vi "zlgcan_demo_EU.vi"() -> ()   [LabVIEW 2018]
doc: "适用的设备：PCI-5010-U、PCI-5020-U、USBCAN-E-U、\nUSBCAN-2E-U、USBCAN-4E-U、USBCAN-8E-U、CANalyst-II+"
uses:
  data_type/ZCAN_Transmit_Data.ctl
  data_type/ZCAN_InitCAN_setting_EU.ctl
panel:
  in  "ZCAN_InitCAN_Setting_EU":T1
  in  "开启CAN":bool
  in  "stop":bool
  in  "?":T2(tab)
  in  "CAN 通道":u32(ring) items=["0", "1"]
  in  "CAN卡型号":u32(ring)=31 items=["PCI-5010-U"=19, "PCI-5020-U"=22, "USBCAN_E_U"=20, "USBCAN_2E_U"=21, "USBCAN-4E-U"=31]
  in  "索引":u32(ring) items=["0", "1", "2", "3", "4", "5", "6", "7", "8"]
  in  "波特率":u32(ring)=500000 items=["1Mbps"=1000000, "800kbps"=800000, "500kbps"=500000, "250kbps"=250000, "125kbps"=125000, "100kbps"=100000, "50kbps"=50000]
  in  "自定义波特率？":bool
  in  "自定义波特率字符输入":string
  in  "工作模式":u8(ring) items=["正常", "只听"]
  out "设备句柄":u32
  out "通道句柄":u32
  out "error out":errorcluster caption="状态"
  in  "帧类型":u32(ring) items=["标准帧", "扩展帧"]
  in  "发送方式":u32(ring) items=["正常发送", "单次发送", "自发自收", "单次自发自收"]
  in  "帧格式":u32(ring) items=["数据帧", "远程帧"]
  out "数据长度":u8=8 max=8
  in  "ID":u32=18 format="0x%08x"
  in  "协议":u32(ring) items=["CAN"]
  in  "数据输入":string="11 22 33 44 55 66 77 88"
  in  "发送":bool
  in  "CAN数据帧数组":T3(array[cluster])
  out "CAN报文显示":string[][](table)
  in  "ZCAN_Transmit_Data":T4
  out "已接收帧数":u32
  # "适用的设备：PCI-5010-U、PCI-5020-U、USBCAN-E-U、\nUSBCAN-2E-U、USBCAN-4E-U"
  # "停止程序前，请先关闭CAN卡"
  # "1. 确保电脑有VC++ 2005/2008/2010/2013运行库（对应32，64位）,微软常用运行库合集，点击下载（35M）。\n    http://manual.zlg.cn/Public/Uploads/2020-06-05/5ed995c271414.zip"
  # "2，如果打开设备失败，可能原因：\n（1）已经打开过一次，没有正常关闭的情况下，继续点击“打开设备”，是无法打开的。\n     需要USB重新拔插，LABVIEW重启（全部关闭），然后再“打开设备”。\n (2) 项目路径不能有中文繁体。"
  # "使用ZCANPro软件波特率计算工具计算"
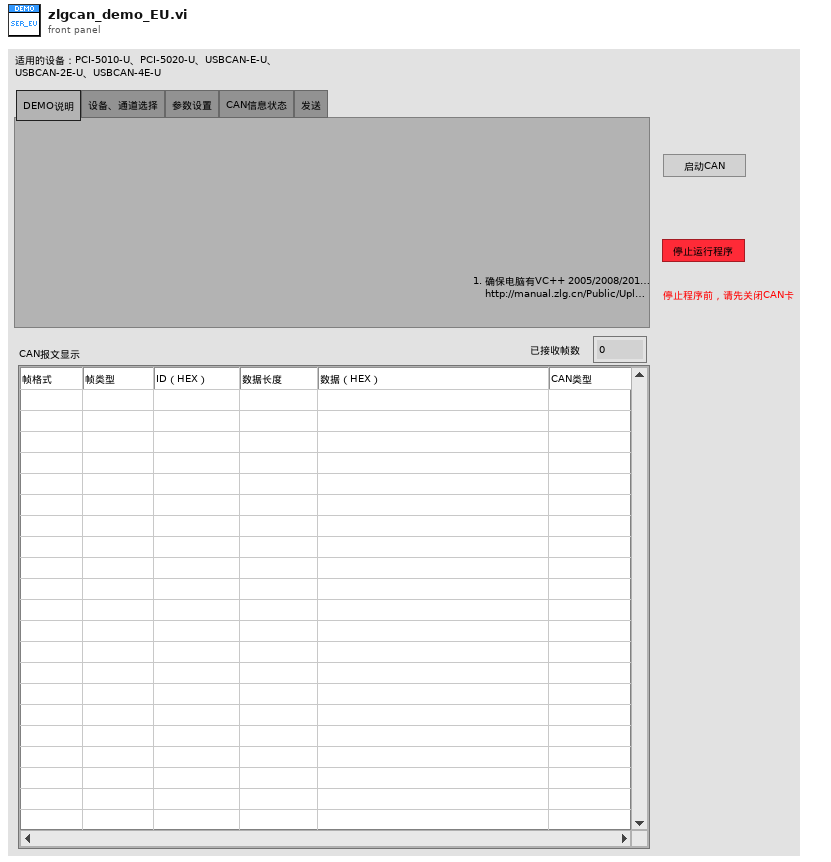
[diagram p1: front panel]
types:
  T1 = typedef "ZCAN_InitCAN_setting_EU.ctl" = cluster{"baudrate":u32, "baud_rate_custom？":bool, "RateCustom":string, "mode":u8}
  T2 = enum32{"DEMO说明", "设备、通道选择", "参数设置", "CAN信息状态", "发送"}
  T3 = cluster{u32, u8, u8, u8, u8, cluster{"[0]":u8, "[1]":u8, "[2]":u8, "[3]":u8, "[4]":u8, "[5]":u8, "[6]":u8, "[7]":u8}, u64}[]
  T4 = typedef "ZCAN_Transmit_Data.ctl" = cluster{"帧类型":u32, "帧格式":u32, "ID":u32, "数据长度":u8, "DATA":cluster{"CAN数据[0]":u8, "CAN数据[1]":u8, "CAN数据[2]":u8, "CAN数据[3]":u8, "CAN数据[4]":u8, "CAN数据[5]":u8, "CAN数据[6]":u8, "CAN数据[7]":u8}, "发送方式":u32}
  T5 = cluster{"[0]":u32, "[1]":u32, "[2]":u32, "[3]":u32, "[4]":u32, "[5]":u32, "[6]":u32, "[7]":u32}
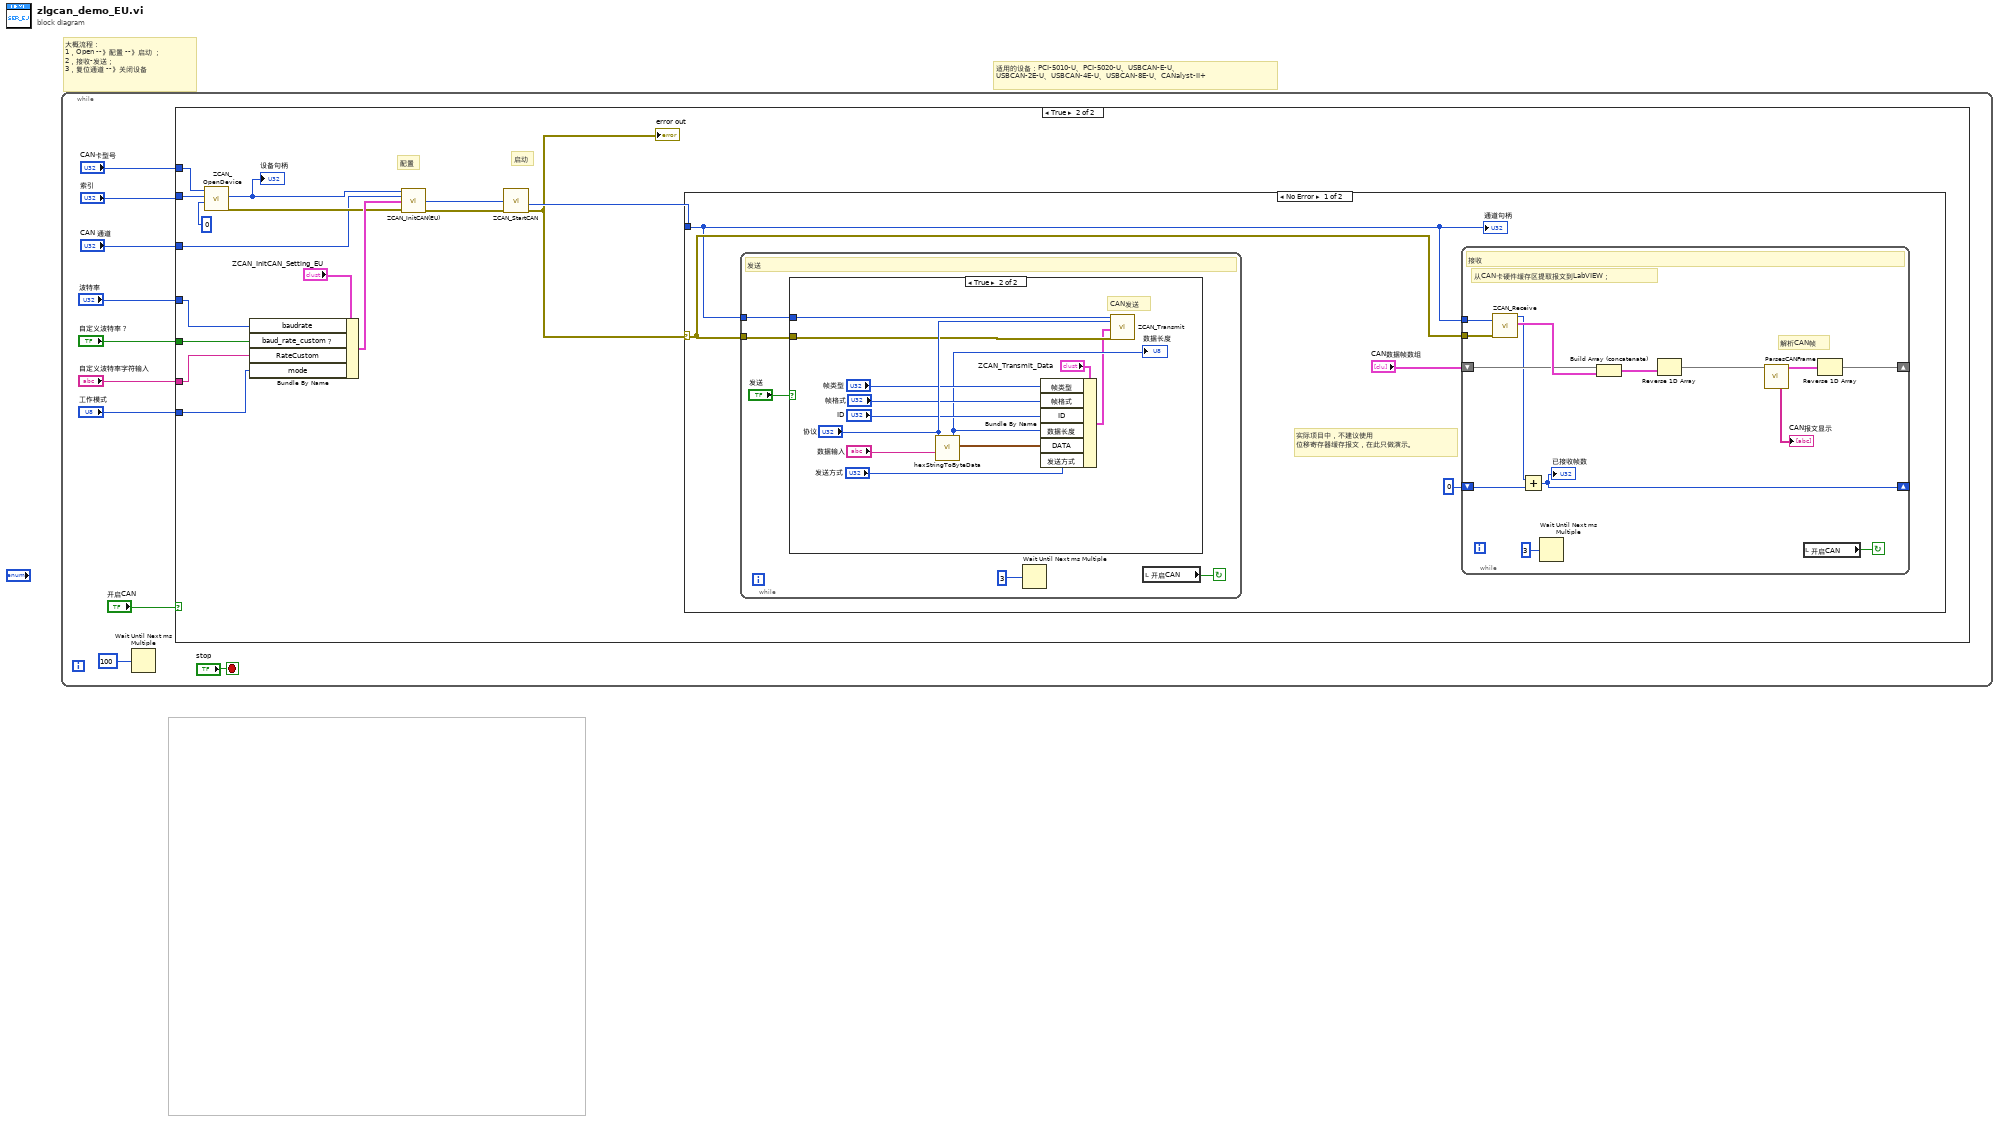
[diagram p0: block diagram]
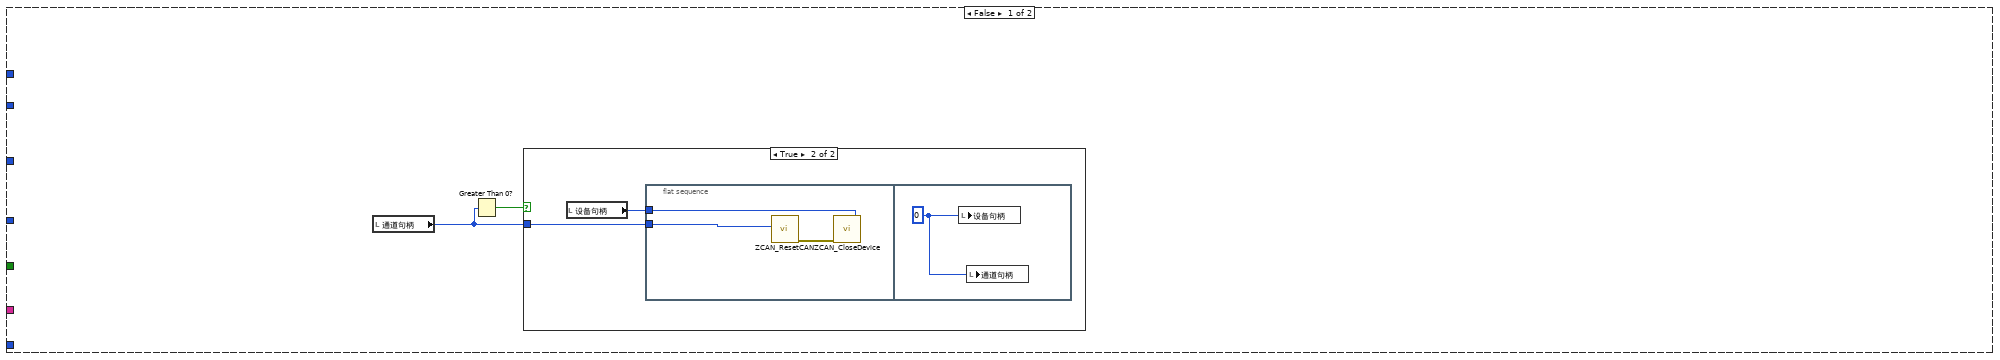
[diagram p2: hidden frame]
diagram:
  # "适用的设备：PCI-5010-U、PCI-5020-U、USBCAN-E-U、\nUSBCAN-2E-U、USBCAN-4E-U、USBCAN-8E-U、CANalyst-II+"
  # "大概流程：\n1，Open --》配置 --》启动 ；\n2，接收-发送；\n3，复位通道 --》关闭设备"
  n1 = while {
    stop <- "stop" stop-if-true
    n2 = Wait Until Next ms Multiple(millisecond multiple=u32 100) -> ()  [unwired: 1 out]
    n3 = case shown="True" "开启CAN" {
      tunnel: "CAN 通道" -> [_ w21]
      tunnel: "CAN卡型号" -> [_ w32]
      tunnel: "索引" -> [_ w33]
      tunnel: "波特率" -> [_ w27]
      tunnel: "自定义波特率？" -> [_ w26]
      tunnel: "自定义波特率字符输入" -> [_ w25]
      tunnel: "工作模式" -> [_ w24]
      frame False {
        # "关闭CAN卡"
        n4 = local read "通道句柄"() -> (w11:u32)
        n5 = Greater Than 0?(x=w11) -> (x > 0?=w12:bool)
        n6 = case shown="True" w12 {
          tunnel: w11 -> [_ w14]
          frame False {
          }
          frame True {
            n7 = local read "设备句柄"() -> (w13:u32)
            n8 = flat-sequence {
              tunnel: w14 -> [w15]
              tunnel: w13 -> [w16]
              frame #0 {
                n9 = call "ZCAN_ResetCAN.vi"("can_handle"=w15) -> ("error out"=w17:errorcluster)  [unwired: 9 in, 1 out]
                n10 = call "ZCAN_CloseDevice.vi"("error in (no error)"=w17, "device_handle"=w16) -> ()  [unwired: 8 in, 2 out]
              }
              frame #1 {
                w18 = u32 0 ("can_index_handle(out)")
                n11 = local write "设备句柄"(w18) -> ()
                n12 = local write "通道句柄"(w18) -> ()
              }
            }
          }
        }
      }
      frame True {
        # "启动"
        # "配置"
        n13 = call "ZCAN_OpenDevice.vi"("reserved"=0, "device_index"=w33, "device_type"=w32) -> ("error out"=w22:errorcluster, "DEVICE_HANDLE"=w23:u32)  [unwired: 7 in]
        "设备句柄" <- w23
        n14 = Bundle By Name(cluster="ZCAN_InitCAN_Setting_EU", "baudrate"=w27, "baud_rate_custom？"=w26, "RateCustom"=w25, "mode"=w24) -> (w29:T1)
        n15 = call "ZCAN_InitCAN(EU).vi"("device_hande"=w23, "can_index"=w21, "ZCAN_InitCAN_Setting_EU"=w29, "error in (no error)"=w22) -> ("can_index_handle"=w20:u32, "error out"=w19:errorcluster)  [unwired: 10 in]
        n16 = call "ZCAN_StartCAN.vi"("error in (no error)"=w19, "can_index_handle"=w20) -> ("error out"=w30:errorcluster, "can_index_handle(out)"=w31:u32)  [unwired: 7 in, 1 out]
        "error out" <- w30
        n17 = case shown="No Error" w30 {
          selector: w30 -> [w37 _]
          tunnel: w31 -> [w36 _]
          frame No Error {
            # "实际项目中，不建议使用\n位移寄存器缓存报文，在此只做演示。"
            n18 = while {
              tunnel: w36 -> [w55]
              tunnel: w37 -> [w53]
              stop <- w54 continue-if-true
              # "发送"
              n19 = case shown="True" "发送" {
                tunnel: w55 -> [_ w62]
                tunnel: w53 -> [_ w63]
                frame False {
                }
                frame True {
                  # "CAN发送"
                  n20 = call "hexStringToByteData.vi"("数据输入"="数据输入", "协议"="协议") -> ("CAN_data"=w59:T5, "字节数"=w64:i32)  [unwired: 7 in, 1 out]
                  "数据长度" <- w64
                  n21 = Bundle By Name(cluster="ZCAN_Transmit_Data", "帧类型"="帧类型", "帧格式"="帧格式", "ID"="ID", "数据长度"=w64, "DATA"=w59, "发送方式"="发送方式") -> (w58:T4)
                  n22 = call "ZCAN_Transmit.vi"("can_index_handle"=w62, "协议"="协议", "ZCAN_Transmit_Data"=w58, "error in (no error)"=w63) -> ()  [unwired: 15 in, 1 out]
                }
              }
              n23 = Wait Until Next ms Multiple(millisecond multiple=u32 3) -> ()  [unwired: 1 out]
              n24 = local read "开启CAN"() -> (w54:bool)
            }
            n25 = while {
              tunnel: w37 -> [w50]
              tunnel: w36 -> [w49]
              shift-right: [w51] -> _
              shift-left: 0 -> [w40]
              shift-right: [w43] -> _
              shift-left: "CAN数据帧数组" -> [w46]
              stop <- w48 continue-if-true
              # "从CAN卡硬件缓存区提取报文到LabVIEW；"
              # "解析CAN帧"
              # "接收"
              n26 = call "ZCAN_Receive.vi"("error in (no error)"=w50, "can_handle"=w49) -> ("CAN数据帧数组"=w47:T3, "Receive_Num"=w41:u32)  [unwired: 2 in, 2 out]
              n27 = Add(x=w41, y=w40) -> (x+y=w51:u32)
              "已接收帧数" <- w51
              n28 = Wait Until Next ms Multiple(millisecond multiple=u32 3) -> ()  [unwired: 1 out]
              n29 = Build Array (concatenate)(w46, w47) -> (w45:T3)
              n30 = Reverse 1D Array(array=w45) -> (reversed array=w42:T3)
              n31 = call "ParsesCANFrame.vi"("CAN数据帧数组"=w42) -> ("CAN数据帧数组(out)"=w44:T3, "CAN报文显示"=→"CAN报文显示":string[][])  [unwired: 9 in]
              n32 = local read "开启CAN"() -> (w48:bool)
              n33 = Reverse 1D Array(array=w44) -> (reversed array=w43:T3)
            }
            "通道句柄" <- w36
          }
          frame Error {
          }
        }
      }
    }
  }
